vi "Actuator fgv.vi"(7 "Enum":T2, 8 "error in (no error)":errorcluster, 10 "Data":variant, 11 "Cluster in":T1={"COM port"="COM4", "Home pos"=0.0, "Speed"=0.5, "Limit stop"=100.0} {"Limit stop" min=0.0 max=150.0 step=0.0001; "Speed" min=0.0001 max=20.0 step=0.0001; "Home pos" min=0.0 max=150.0 step=0.0001}) -> (0 "error out":errorcluster, 3 "Cluster out":T1={"COM port"="COM4", "Home pos"=0.0, "Speed"=0.5, "Limit stop"=100.0} {"Limit stop" min=0.0 max=150.0 step=0.0001; "Speed" min=0.0001 max=20.0 step=0.0001; "Home pos" min=0.0 max=150.0 step=0.0001})   [LabVIEW 2016]
uses:
  Controls/Actuator fgv modes.ctl
  Controls/Default settings.ctl
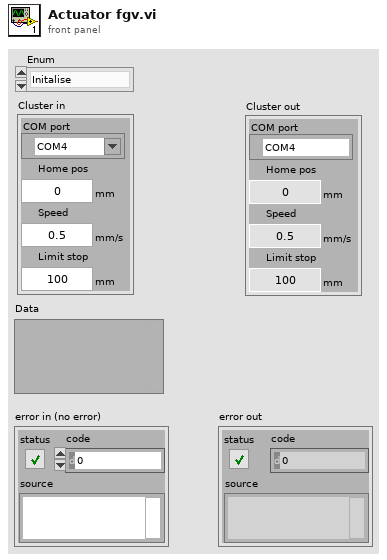
[diagram p1: front panel]
types:
  T1 = typedef "Default settings.ctl" = cluster{"COM port":refnum<visa-resource-name>, "Home pos":dbl, "Speed":dbl, "Limit stop":dbl}
  T2 = typedef "Actuator fgv modes.ctl" = enum16{"Initalise", "COM", "Limit", "Speed", "Home", "Get"}
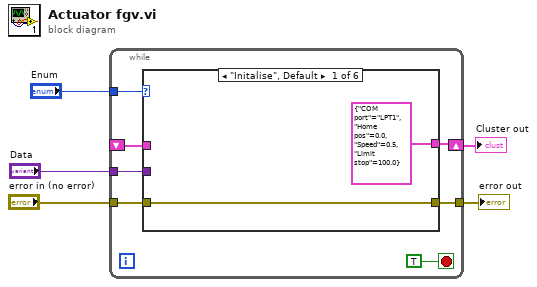
[diagram p0: block diagram]
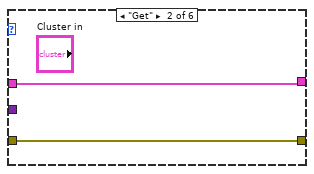
[diagram p2: hidden frame]
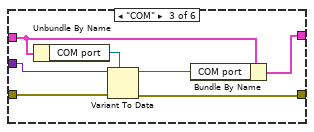
[diagram p3: hidden frame]
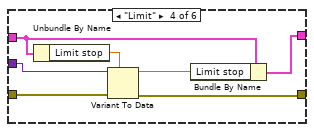
[diagram p4: hidden frame]
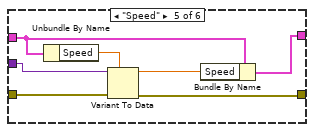
[diagram p5: hidden frame]
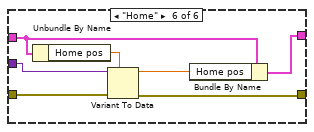
[diagram p6: hidden frame]
diagram:
  n1 = while {
    shift-right: [w10] -> w2
    shift-left: _ -> [w7]
    tunnel: "Enum" -> [w11]
    tunnel: "error in (no error)" -> [w9]
    tunnel: [w8] -> w3
    tunnel: "Data" -> [w6]
    stop <- TRUE stop-if-true
    n2 = case shown="\"Initalise\", Default" w11 {
      tunnel: [T1 {"COM port"="LPT1", "Home pos"=0.0, "Speed"=0.5, "Limit stop"=100.0} ("Cluster in") w15 w20 w27 w34 w41] -> w10
      tunnel: w9 -> [w13 w16 w23 w30 w37 w44]
      tunnel: [w13 w16 w17 w24 w31 w38] -> w8
      tunnel: w7 -> [_ w15 w19 w26 w33 w40]
      tunnel: w6 -> [_ _ w22 w29 w36 w43]
      frame "Initalise", Default {
      }
      frame "Get" {
      }
      frame "COM" {
        n3 = Unbundle By Name(w19) -> ("COM port"=w21:refnum<visa-resource-name>)
        n4 = Variant To Data(error in=w23, type=w21, Variant=w22) -> (data=w18:refnum<visa-resource-name>, error out=w17:errorcluster)
        n5 = Bundle By Name(cluster=w19, "COM port"=w18) -> (w20:T1)
      }
      frame "Limit" {
        n6 = Unbundle By Name(w26) -> ("Limit stop"=w28:dbl)
        n7 = Variant To Data(error in=w30, type=w28, Variant=w29) -> (data=w25:dbl, error out=w24:errorcluster)
        n8 = Bundle By Name(cluster=w26, "Limit stop"=w25) -> (w27:T1)
      }
      frame "Speed" {
        n9 = Unbundle By Name(w33) -> ("Speed"=w35:dbl)
        n10 = Variant To Data(error in=w37, type=w35, Variant=w36) -> (data=w32:dbl, error out=w31:errorcluster)
        n11 = Bundle By Name(cluster=w33, "Speed"=w32) -> (w34:T1)
      }
      frame "Home" {
        n12 = Unbundle By Name(w40) -> ("Home pos"=w42:dbl)
        n13 = Variant To Data(error in=w44, type=w42, Variant=w43) -> (data=w39:dbl, error out=w38:errorcluster)
        n14 = Bundle By Name(cluster=w40, "Home pos"=w39) -> (w41:T1)
      }
    }
  }
  "error out" <- w3
  "Cluster out" <- w2
